vi "Write Device Name.vi"(8 "error in (no error)":errorcluster, 10 "Device Name":string, 11 "Hardware in":refnum<class "Hardware.lvclass">) -> (0 "error out":errorcluster, 3 "Hardware out":refnum<class "Hardware.lvclass">)   [LabVIEW 2026, in "TALOS.lvlib" / "Classes.lvlib" / "Hardware.lvclass"]
uses:
  Hardware.lvclass
  Hardware.lvclass/Hardware.ctl
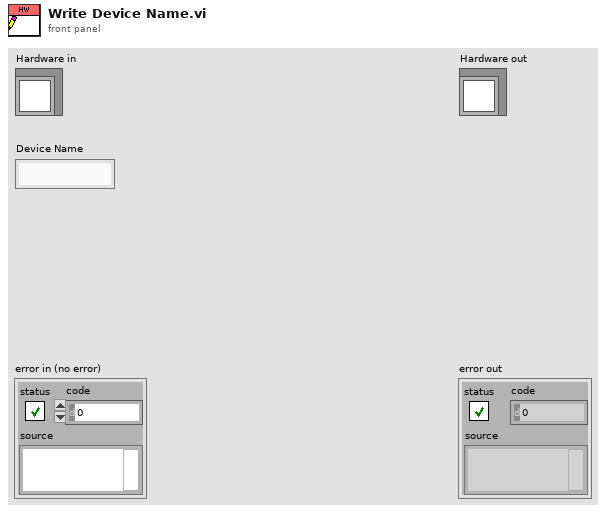
[diagram p1: front panel]
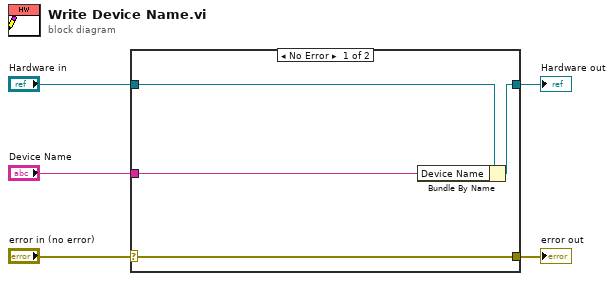
[diagram p0: block diagram]
diagram:
  n1 = case shown="No Error" "error in (no error)" {
    selector: "error in (no error)" -> [w9 w10]
    tunnel: [w9 w10] -> w4
    tunnel: [w7 w11] -> w2
    tunnel: "Hardware in" -> [w8 w11]
    tunnel: "Device Name" -> [w6 _]
    frame No Error {
      n2 = Bundle By Name(cluster=w8, "Device Name"=w6) -> (w7:refnum<class "Hardware.lvclass">)
    }
    frame Error {
    }
  }
  "error out" <- w4
  "Hardware out" <- w2
